vi "get GEECS network card IP.vi"() -> (3 "GEECS computer IP":string)   [LabVIEW 2020]
uses:
  MySQL/Preset Query Enum.ctl
  <userlib>/_OpenG.lib/array/array.llb/Remove Duplicates from 1D Array (String)__ogtk.vi
  <userlib>/_OpenG.lib/array/array.llb/Search 1D Array (String)__ogtk.vi
panel:
  out "element":string
  out "Network Card IPs 1st 3 segments":string[](array[string])
  out "Unique GEECS IPs 1st 3 segements":string[](array[string])
  out "IP adresses":string[](array[string])
  out "Indices of Elements":i32[](array[numeric])
  out "error out":errorcluster
  in  "error in (no error)":errorcluster
  out "All IPs":string[](array[string])
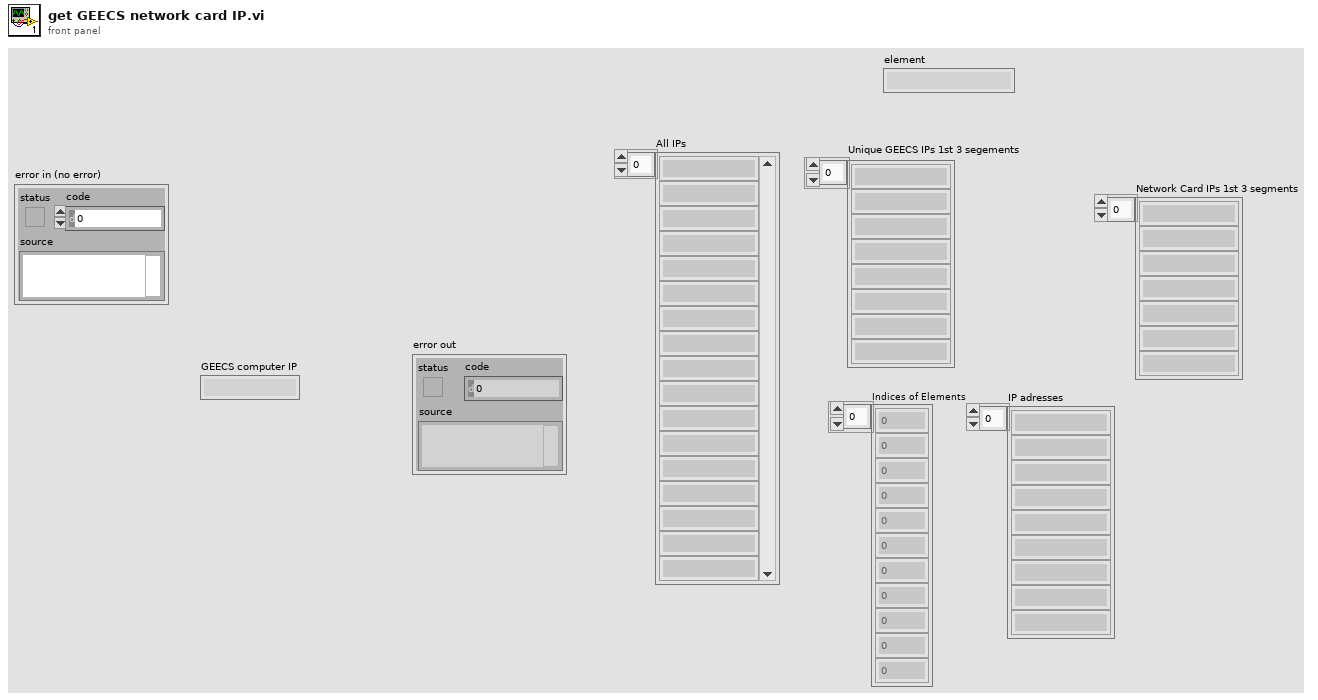
[diagram p1: front panel]
types:
  T1 = typedef "Preset Query Enum.ctl" = enum16{"Get Locations", "Get all IPs and MACs", "Get classes", "Get expt variables to set at scanstart for particular device", "Get expt devices and variables with start values", "Get expt devices and variables (with data to get)", "Get expt devices with data to get", "Get Expt devices and GUIs", "Get all devices basic properties", "Get Virtual Devices Core Info", "Get Expt names", "Get experiment basic properties", "Get experiment alarm variables", "Get MC Ports", "Get device network comm port", "Get devicetype lvclass path", "Get basic device properties", "Get Init Order", "Get all setable variables of a device", "Get device variable aliases", "Get force values of all settable variables", "Get all variables of a devicetype", "Get all variables of a device", "Get plotter details", "Get Saved Scans", "Get Scan Info", "GetGeneralGUIs", "Get expt for plotter", "Get plotter IDs from expt", "Get all devices", "Get all Virtual Devices", "Get all aliases", "Get variable and device info for Virtual Device", "GetItemLocatorIP", "Get IPs for GUIs", "Get DeviceType from Device", "GetLocalPortRange", "GetDevicePresetVariables", "Get Device Configuration", "GetAllPresetNames", "GetAllConfigurationNames", "GetPresetDeviceNames", "GetDeviceAliases", "GetDevicesOfClass"}
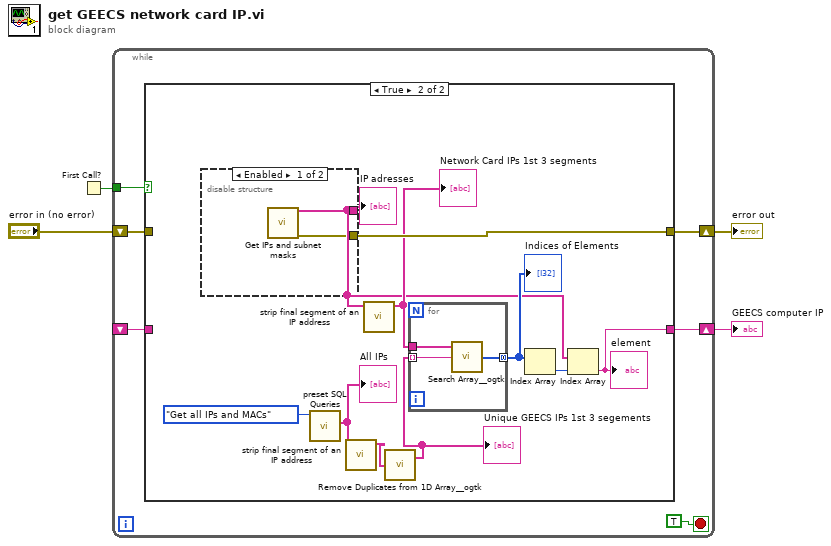
[diagram p0: block diagram]
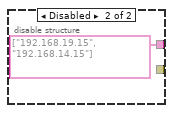
[diagram p3: hidden frame]
diagram:
  n1 = First Call?() -> (First Call?: T/F=w1:bool)
  n2 = while {
    shift-right: [w8] -> w2
    shift-left: "error in (no error)" -> [w10]
    shift-right: [w9] -> w3
    shift-left: _ -> [w6]
    tunnel: w1 -> [w7]
    stop <- TRUE stop-if-true
    n3 = case shown="True" w7 {
      tunnel: w10 -> [w11 _]
      tunnel: [w12 w15] -> w9
      tunnel: [w11 w22] -> w8
      tunnel: w6 -> [w12 _]
      frame False {
      }
      frame True {
        n4 = disable-structure shown="Enabled" {
          disable-tunnel: [w24 _] -> w22
          disable-tunnel: [w23 string[] ["192.168.19.15", "192.168.14.15"] ("1st column 1st data")] -> w16
          frame Enabled {
            n5 = call "Get IPs and subnet masks.vi"() -> ("IP adresses"=w23:string[], "error out"=w24:errorcluster)  [unwired: 11 in, 3 out]
          }
          frame Disabled {
          }
        }
        "IP adresses" <- w16
        n6 = call "preset SQL Queries.vi"("Preset Query"=Preset_Query_Enum."Get all IPs and MACs") -> ("1st column 1st data"=w19:string[])  [unwired: 8 in, 2 out]
        "All IPs" <- w19
        n7 = call "strip final segment of an IP address.vi"("1st column 1st data"=w19) -> ("Output Array"=w14:string[])  [unwired: 10 in]
        n8 = call "strip final segment of an IP address.vi"("1st column 1st data"=w16) -> ("Output Array"=w17:string[])  [unwired: 10 in]
        "Network Card IPs 1st 3 segments" <- w17
        n9 = call-poly <userlib>:"Remove Duplicates from 1D Array__ogtk.vi"("Input Array"=w14) -> ("Output Array"=w13:string[])  [unwired: 1 out]
        "Unique GEECS IPs 1st 3 segements" <- w13
        n10 = for {
          tunnel: [w28] -> w20 mode=concatenating
          tunnel: w13 -> [w26] mode=indexing
          tunnel: w17 -> [w27]
          n11 = call-poly <userlib>:"Search Array__ogtk.vi"("Array"=w27, "Element Data"=w26) -> ("Indices of Elements"=w28:i32[])  [unwired: 7 in]
        }
        "Indices of Elements" <- w20
        n12 = Index Array(array=w20) -> (element=w18:i32)  [unwired: 1 in]
        n13 = Index Array(array=w16, index=w18) -> (element=w15:string)
        "element" <- w15
      }
    }
  }
  "GEECS computer IP" <- w3
  "error out" <- w2
